vi "SFCSetting.vi"() -> (2 "SFC Setting Out":bool)   [LabVIEW 2009]
panel:
  in  "SFC Setting":bool
  in  "OK Button":bool
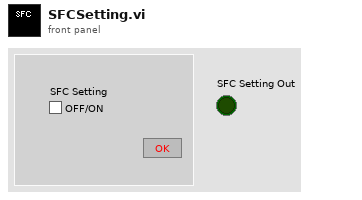
[diagram p1: front panel]
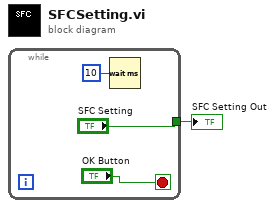
[diagram p0: block diagram]
diagram:
  n1 = while {
    tunnel: ["SFC Setting"] -> w1
    stop <- "OK Button" stop-if-true
    n2 = Wait (ms)(milliseconds to wait=u32 10) -> ()  [unwired: 1 out]
  }
  "SFC Setting Out" <- w1
